vi "Copy Graph to Clipboard.vi"(8 "error in (no error)":errorcluster, 11 "Graph Data":T1={"UI References"={"Stop Ref"=refnum, "Save Ref"=refnum, "Open Ref"=refnum, "Export Ref"=refnum, "Acquire Ref"=refnum, "Configure Ref"=refnum, "Graph Ref"=refnum, "Clear Ref"=refnum, "Analyze Ref"=refnum, "Status Ref"=refnum, "Snapshot Ref"=refnum}, "Graph Data"={"Data"=[], "Annotation List"=[], "Cursor List"=[], "Analysis Data"=[]}, "User Specified"={"Hardware Configuration"={"Physical Channel"="", "Maximum Input"=0.0, "Minimum Input"=0.0, "Sample Rate"=0.0, "Number of Samples"=0}, "Analysis Configuration"={"Statistics"=TRUE}, "New Data Behavior"=enum."Replace"}}) -> (0 "error out":errorcluster)   [LabVIEW 2018]
doc: "Copies an image of the graph to the clipboard."
uses:
  controls/Data.ctl
  controls/UI References.ctl
  controls/Graph Data.ctl
  <vilib>/Utility/miscctls.llb/LVAnnotationListTypeDef.ctl
  <vilib>/Utility/miscctls.llb/LVCursorListTypeDef.ctl
  controls/User Specified Data.ctl
  controls/HW Configuration.ctl
  controls/Analysis Configuration.ctl
  controls/New Data Behavior.ctl
panel:
  # "(Scroll up to see large data cluster)"
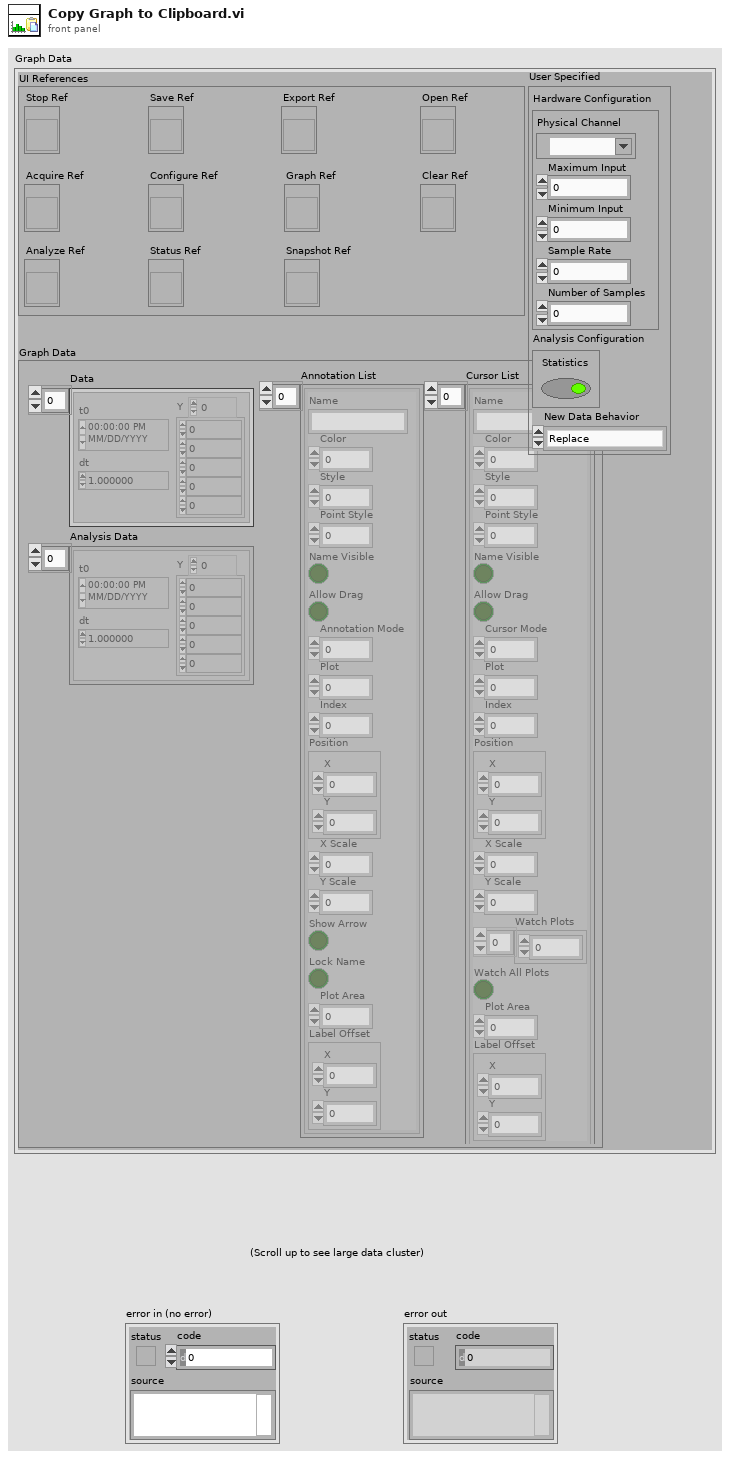
[diagram p1: front panel]
types:
  T1 = typedef "Data.ctl" = cluster{"UI References":T2, "Graph Data":T3, "User Specified":T6}
  T2 = typedef "UI References.ctl" = cluster{"Stop Ref":refnum<vi>, "Save Ref":refnum<vi>, "Open Ref":refnum<vi>, "Export Ref":refnum<vi>, "Acquire Ref":refnum<vi>, "Configure Ref":refnum<vi>, "Graph Ref":refnum<vi>, "Clear Ref":refnum<vi>, "Analyze Ref":refnum<vi>, "Status Ref":refnum<vi>, "Snapshot Ref":refnum<vi>}
  T3 = typedef "Graph Data.ctl" = cluster{"Data":waveform(dbl)[], "Annotation List":T4, "Cursor List":T5, "Analysis Data":waveform(dbl)[]}
  T4 = typedef "LVAnnotationListTypeDef.ctl" = cluster{"Name":string, "Color":u32, "Style":u8, "Point Style":u8, "Name Visible":bool, "Allow Drag":bool, "Annotation Mode":u32, "Plot":i32, "Index":i32, "Position":cluster{"X":dbl, "Y":dbl}, "X Scale":u32, "Y Scale":u32, "Show Arrow":bool, "Lock Name":bool, "Plot Area":i32, "Label Offset":cluster{"X":dbl, "Y":dbl}}[]
  T5 = typedef "LVCursorListTypeDef.ctl" = cluster{"Name":string, "Color":u32, "Style":u8, "Point Style":u8, "Name Visible":bool, "Allow Drag":bool, "Cursor Mode":u32, "Plot":i32, "Index":i32, "Position":cluster{"X":dbl, "Y":dbl}, "X Scale":u32, "Y Scale":u32, "Watch Plots":i32[], "Watch All Plots":bool, "Plot Area":i32, "Label Offset":cluster{"X":dbl, "Y":dbl}}[]
  T6 = typedef "User Specified Data.ctl" = cluster{"Hardware Configuration":T7, "Analysis Configuration":T8, "New Data Behavior":T9}
  T7 = typedef "HW Configuration.ctl" = cluster{"Physical Channel":tag, "Maximum Input":dbl, "Minimum Input":dbl, "Sample Rate":dbl, "Number of Samples":i32}
  T8 = typedef "Analysis Configuration.ctl" = cluster{"Statistics":bool}
  T9 = typedef "New Data Behavior.ctl" = enum16{"Replace", "Overlay", "Append"}
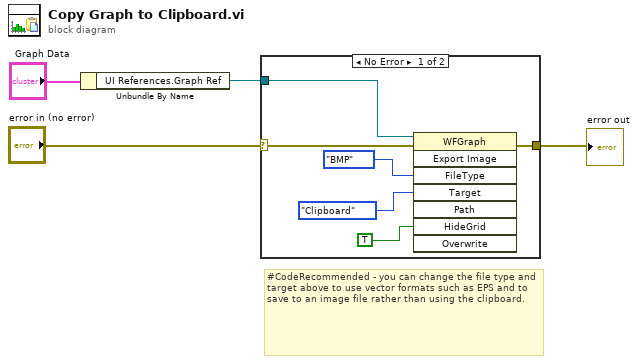
[diagram p0: block diagram]
diagram:
  # "#CodeRecommended - you can change the file type and target above to use vector formats such as EPS and to save to an image file rather than using the clipboard."
  n1 = Unbundle By Name("Graph Data") -> ("UI References.Graph Ref"=w3:refnum<vi>)
  n2 = case shown="No Error" "error in (no error)" {
    selector: "error in (no error)" -> [w5 w11]
    tunnel: w3 -> [w10 _]
    tunnel: [w6 w11] -> w2
    frame No Error {
      n3 = invoke class="WFGraph" method="Export Image"(reference=w10, error in=w5, "FileType"=enum32{"BMP", "EPS", "EMF", "PICT"}."BMP" ("File Type"), "Target"=enum32{"File", "Clipboard"}."Clipboard", "HideGrid"=TRUE ("Hide Grid")) -> (error out=w6:errorcluster)  [unwired: 3 in, 7 out]
    }
    frame Error {
    }
  }
  "error out" <- w2
